vi "Home Elevator.vi"(11 "Execute?":bool) -> (3 "Done":bool)   [LabVIEW 2012]
uses:
  Globals/Useful Values.vi
  Globals/Shooter Elevation Positons.vi
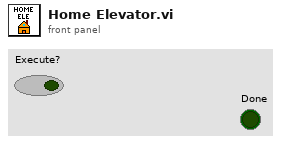
[diagram p1: front panel]
types:
  T1 = typedef "WPI_AnalogChannelDevRef.ctl" = cluster{"DevStatus":errorcluster, "Analog Module":T2, "Analog Channel":T3}
  T2 = typedef "FPGA_TypedefAnalogModule.ctl" = enum16{"Analog Module 1", "Analog Module 2"}
  T3 = typedef "FPGA_AIChannel.ctl" = enum8{"AI 1", "AI 2", "AI 3", "AI 4", "AI 5", "AI 6", "AI 7", "AI 8", "Invalid"}
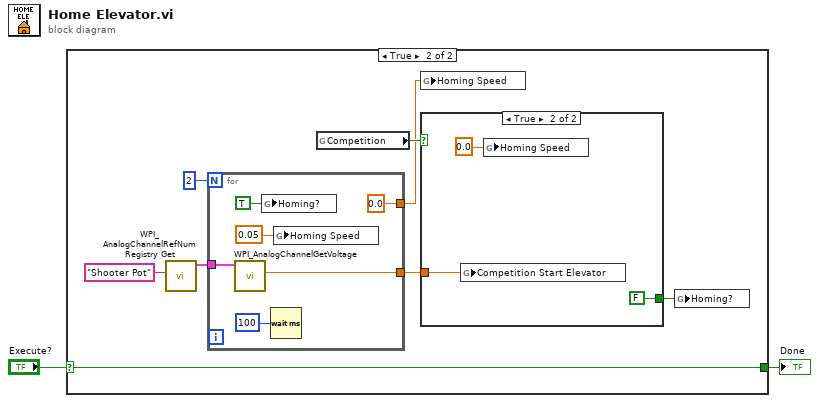
[diagram p0: block diagram]
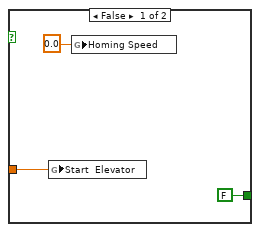
[diagram p3: hidden frame]
diagram:
  n1 = case shown="True" "Execute?" {
    selector: "Execute?" -> [w3 w6]
    tunnel: [w3 w6] -> w1
    frame False {
    }
    frame True {
      n2 = call <vilib>:"WPI_AnalogChannelRefNum Registry Get.vi"("refnum name"="Shooter Pot") -> ("AIDeviceRef"=w7:T1)  [unwired: 9 in, 1 out]
      n3 = for {
        N: 2 -> [_]
        tunnel: w7 -> [w23]
        tunnel: [w21] -> w10
        tunnel: [0.0 ("Homing Speed")] -> w5
        n4 = call <vilib>:"WPI_AnalogChannelGetVoltage.vi"("AIDeviceRef"=w23) -> ("Voltage"=w21:dbl)  [unwired: 8 in, 2 out]
        n5 = global write "Useful Values.vi" "Homing?"(TRUE ("Homing?")) -> ()
        n6 = Wait (ms)(milliseconds to wait=u32 100) -> ()  [unwired: 1 out]
        n7 = global write "Useful Values.vi" "Homing Speed"(0.05 ("Homing Speed")) -> ()
      }
      n8 = global read "Useful Values.vi" "Competition"() -> (w9:bool)
      n9 = global write "Useful Values.vi" "Homing Speed"(w5) -> ()
      n10 = case shown="True" w9 {
        tunnel: w10 -> [w14 w17]
        tunnel: [FALSE ("Homing?") FALSE ("Homing?")] -> w4
        frame False {
          n11 = global write "Shooter Elevation Positons.vi" "Start  Elevator"(w14) -> ()
          n12 = global write "Useful Values.vi" "Homing Speed"(0.0 ("Homing Speed")) -> ()
        }
        frame True {
          n13 = global write "Shooter Elevation Positons.vi" "Competition Start Elevator"(w17) -> ()
          n14 = global write "Useful Values.vi" "Homing Speed"(0.0 ("Homing Speed")) -> ()
        }
      }
      n15 = global write "Useful Values.vi" "Homing?"(w4) -> ()
    }
  }
  "Done" <- w1
